vi "EditorMethod runPyProcess.vi"(5 "replace?(T)":bool=TRUE, 7 "func":T1, 8 "error in (no error)":errorcluster, 10 "newScriptCode":string, 11 "dataParam":T3) -> (0 "error out":errorcluster={"status"=FALSE, "code"=0, "source"="codeError source : \ncodeError message : \ncodeError line : "}, 2 "pyCode":string, 3 "newSigInfo":T2, 4 "showMsg":string[](array[string]))   [LabVIEW 2018]
uses:
  ctl/editScriptState.ctl
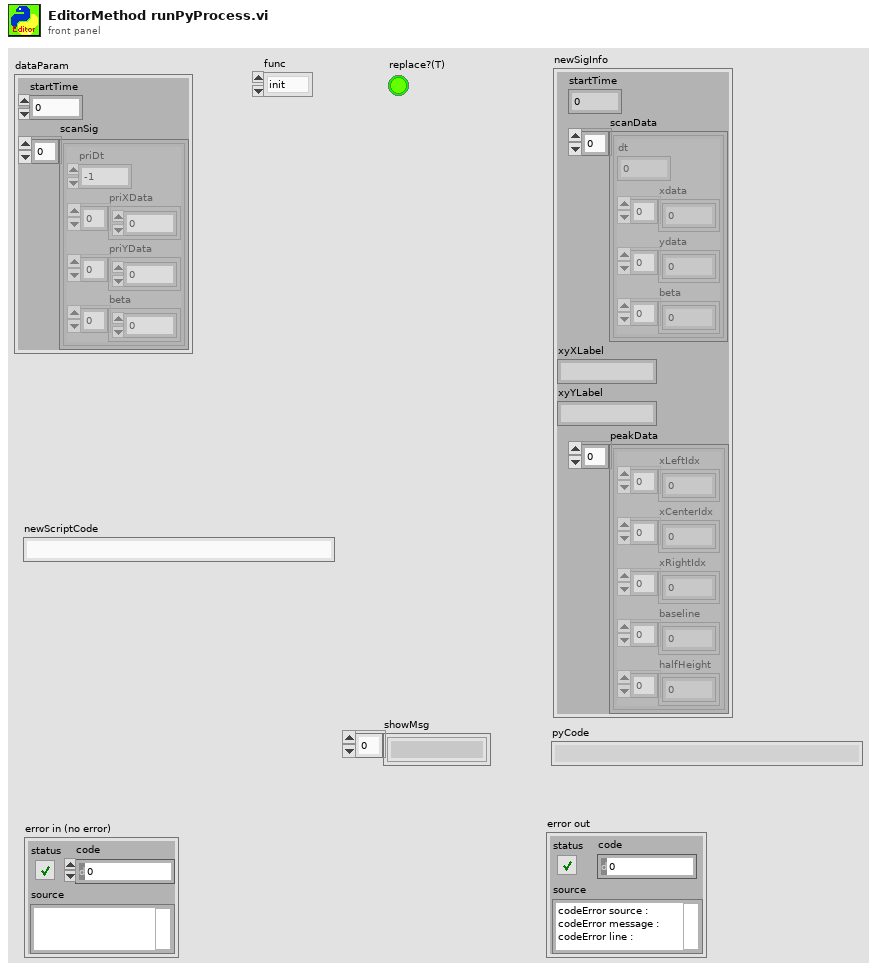
[diagram p1: front panel]
types:
  T1 = typedef "editScriptState.ctl" = enum16{"init", "loadScript", "newScript", "runScript", "close"}
  T2 = cluster{"startTime":dbl, "scanData":cluster{"dt":dbl, "xdata":dbl[], "ydata":sgl[], "beta":dbl[]}[], "xyXLabel":string, "xyYLabel":string, "peakData":cluster{"xLeftIdx":u32[], "xCenterIdx":u32[], "xRightIdx":u32[], "baseline":sgl[], "halfHeight":dbl[]}[]}
  T3 = cluster{"startTime":dbl, "scanSig":cluster{"priDt":dbl, "priXData":dbl[], "priYData":sgl[], "beta":dbl[]}[]}
  T4 = enum16{"open", "replace", "create", "open or create", "replace or create", "replace or create with confirmation"}
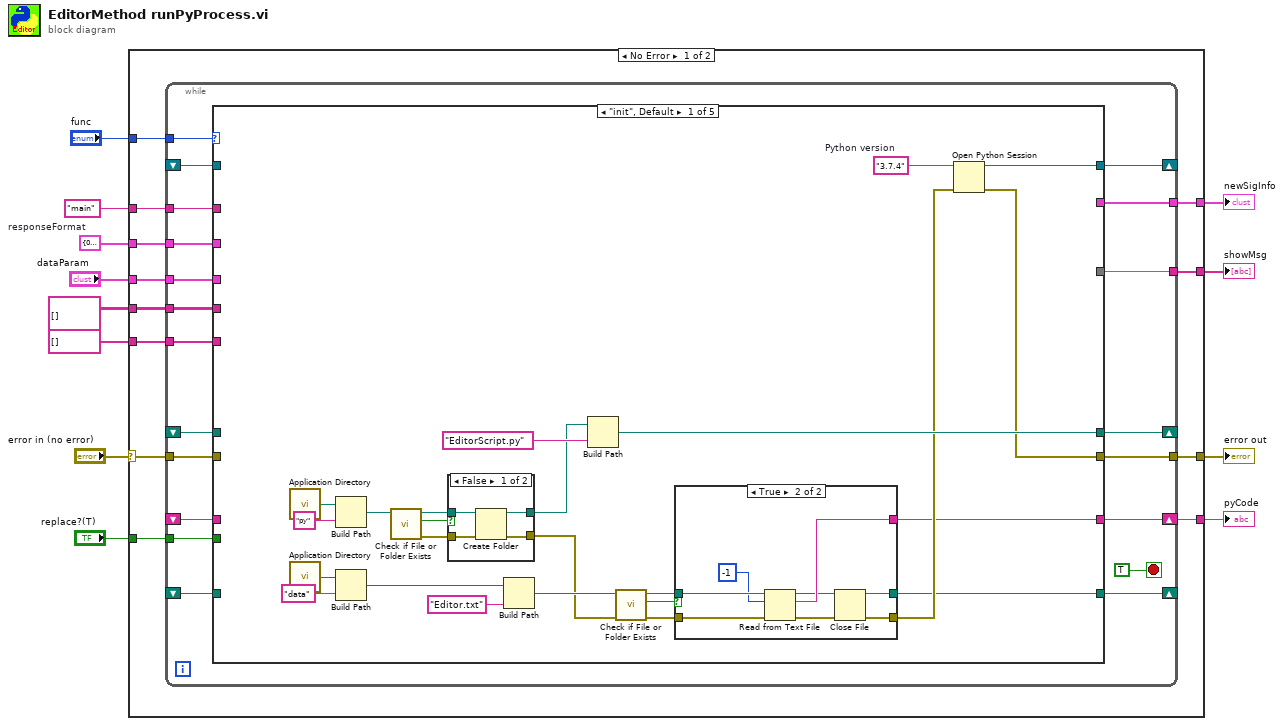
[diagram p0: block diagram]
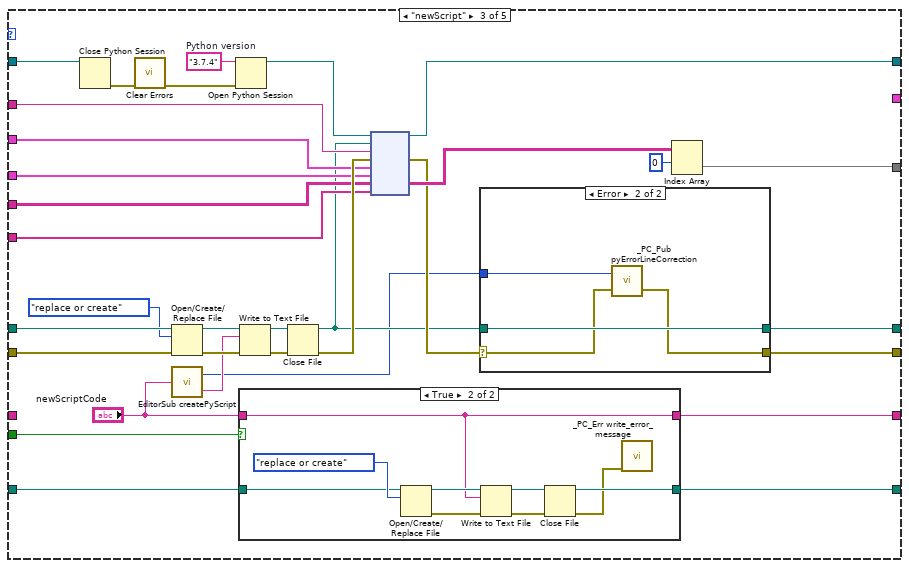
[diagram p5: hidden frame]
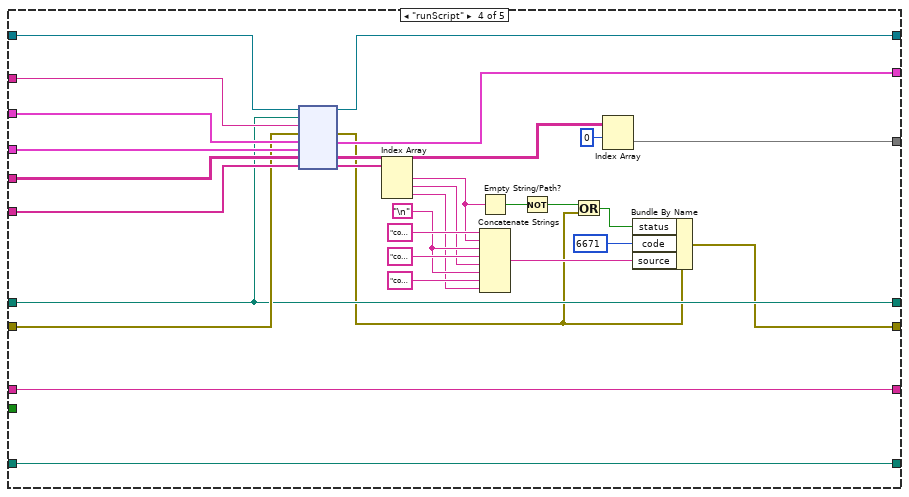
[diagram p8: hidden frame]
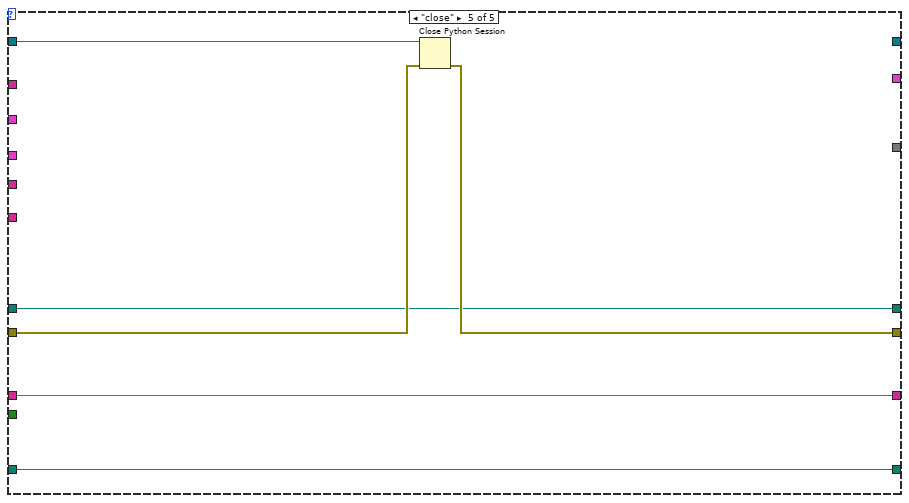
[diagram p9: hidden frame]
diagram:
  w3 = T2 {"startTime"=0.0, "scanData"=[], "xyXLabel"="", "xyYLabel"="", "peakData"=[]}  # responseFormat
  n1 = case shown="No Error" "error in (no error)" {
    selector: "error in (no error)" -> [w19 w176]
    tunnel: "func" -> [w24 _]
    tunnel: [w23 _] -> w12
    tunnel: [w22 _] -> w2
    tunnel: [w21 w176] -> w11
    tunnel: "dataParam" -> [w20 _]
    tunnel: "replace?(T)" -> [w18 _]
    tunnel: [w17 _] -> w7
    tunnel: w3 -> [w16 _]
    tunnel: string[][] [] -> [w15 _]
    tunnel: string[] [] -> [w14 _]
    tunnel: "main" ("function name") -> [w13 _]
    frame No Error {
      n2 = while {
        tunnel: w24 -> [w44]
        shift-right: [w43] -> _
        shift-left: _ -> [w42]
        shift-right: [w41] -> _
        shift-left: _ -> [w40]
        tunnel: [w37] -> w22
        tunnel: w19 -> [w39]
        tunnel: [w35] -> w21
        tunnel: w20 -> [w34]
        tunnel: w18 -> [w33]
        tunnel: [w32] -> w17
        shift-right: [w38] -> w23
        shift-left: _ -> [w31]
        shift-right: [w30] -> _
        shift-left: _ -> [w29]
        tunnel: w16 -> [w28]
        tunnel: w15 -> [w27]
        tunnel: w14 -> [w26]
        tunnel: w13 -> [w25]
        stop <- TRUE stop-if-true
        n3 = case shown="\"init\", Default" w44 {
          tunnel: [w67 w89 w115 w169 _] -> w43
          tunnel: w42 -> [_ w89 w112 w160 w175]
          tunnel: [w58 w86 w93 w147 w173] -> w35
          tunnel: [w59 w88 w94 w148 w172] -> w41
          tunnel: w40 -> [_ w88 w121 w148 w172]
          tunnel: w39 -> [_ w86 w120 w149 w174]
          tunnel: [w45 w87 w122 w155 w170] -> w38
          tunnel: [_ _ _ w162 _] -> w37
          tunnel: w34 -> [_ _ w101 w161 _]
          tunnel: w33 -> [_ _ w113 _ _]
          tunnel: [_ _ w96 w157 _] -> w32
          tunnel: w31 -> [_ w87 _ w155 w170]
          tunnel: [w46 w85 w105 w154 w171] -> w30
          tunnel: w29 -> [_ w85 w106 w154 w171]
          tunnel: w28 -> [_ _ w102 w153 _]
          tunnel: w27 -> [_ _ w100 w151 _]
          tunnel: w26 -> [_ _ w99 w150 _]
          tunnel: w25 -> [_ _ w98 w152 _]
          frame "init", Default {
            w68 = "3.7.4"  # Python version
            n4 = call <vilib>:"Application Directory.vi"() -> ("Application Directory"=w65:path)
            n5 = call <vilib>:"Application Directory.vi"() -> ("Application Directory"=w54:path)
            n6 = Build Path(base path=w65, name or relative path="py") -> (appended path=w56:path)
            n7 = Build Path(base path=w54, name or relative path="data") -> (appended path=w53:path)
            n8 = call <vilib>:"Check if File or Folder Exists.vi"("path"=w56) -> ("error out"=w62:errorcluster, "file or folder exists?"=w64:bool, "dup path"=w63:path)  [unwired: 8 in]
            n9 = case shown="False" w64 {
              tunnel: w63 -> [w82 w84]
              tunnel: w62 -> [w81 w83]
              tunnel: [w80 w84] -> w60
              tunnel: [w79 w83] -> w48
              frame False {
                n10 = Create Folder(path (use dialog)=w82, error in=w81) -> (created path=w80:path, error out=w79:errorcluster)  [unwired: 1 in, 1 out]
              }
              frame True {
              }
            }
            n11 = Build Path(base path=w53, name or relative path="Editor.txt") -> (appended path=w49:path)
            n12 = Build Path(base path=w60, name or relative path="EditorScript.py") -> (appended path=w59:path)
            n13 = call <vilib>:"Check if File or Folder Exists.vi"("error in (no error)"=w48, "path"=w49) -> ("error out"=w50:errorcluster, "file or folder exists?"=w51:bool, "dup path"=w52:path)  [unwired: 7 in]
            n14 = case shown="True" w51 {
              tunnel: w52 -> [w70 w78]
              tunnel: w50 -> [w69 w77]
              tunnel: [_ w76] -> w45
              tunnel: [w70 w72] -> w46
              tunnel: [w69 w71] -> w47
              frame False {
              }
              frame True {
                n15 = Read from Text File(file (use dialog)=w78, count=-1, error in=w77) -> (refnum out=w73:refnum<file>, text=w76:string, error out=w74:errorcluster)  [unwired: 1 in, 1 out]
                n16 = Close File(refnum=w73, error in=w74) -> (path=w72:path, error out=w71:errorcluster)
              }
            }
            n17 = Open Python Session(python version=w68, 3:w47) -> (session out=w67:refnum<k35>, error out=w58:errorcluster)  [unwired: 1 in]
          }
          frame "loadScript" {
          }
          frame "newScript" {
            w109 = "3.7.4"  # Python version
            n18 = Close Python Session(session in=w112) -> (11:w111:errorcluster)  [unwired: 1 in]
            n19 = call <vilib>:"Clear Errors.vi"("error in (no error)"=w111) -> ("error out"=w110:errorcluster)  [unwired: 5 in, 1 out]
            n20 = Open/Create/Replace File(file path (use dialog)=w121, error in=w120, operation (0:open)=T4."replace or create") -> (refnum out=w119:refnum<file>, error out=w118:errorcluster)  [unwired: 3 in, 1 out]
            n21 = call "EditorSub createPyScript.vi"("newScriptCode"="newScriptCode") -> ("scriptStartIdx"=w90:i32, "pyCode"=w103:string)
            n22 = Open Python Session(python version=w109, 3:w110) -> (session out=w108:refnum<k35>)  [unwired: 1 in, 1 out]
            n23 = case shown="True" w113 {
              tunnel: "newScriptCode" -> [w130 w132]
              tunnel: [w130 w132] -> w122
              tunnel: w106 -> [w129 w134]
              tunnel: [w129 w133] -> w105
              frame False {
              }
              frame True {
                n24 = Open/Create/Replace File(file path (use dialog)=w134, operation (0:open)=T4."replace or create") -> (refnum out=w136:refnum<file>, error out=w138:errorcluster)  [unwired: 4 in, 1 out]
                n25 = Write to Text File(file (use dialog)=w136, text=w132, error in=w138) -> (refnum out=w137:refnum<file>, error out=w139:errorcluster)  [unwired: 1 in, 1 out]
                n26 = Close File(refnum=w137, error in=w139) -> (path=w133:path, error out=w131:errorcluster)
                n27 = call "_PC_Err write_error_message.vi"("error in"=w131) -> ()  [unwired: 10 in, 1 out]
              }
            }
            n28 = Write to Text File(file (use dialog)=w119, text=w103, error in=w118) -> (refnum out=w117:refnum<file>, error out=w116:errorcluster)  [unwired: 1 in, 1 out]
            n29 = Close File(refnum=w117, error in=w116) -> (path=w91:path, error out=w107:errorcluster)
            n30 = node(w108, w91, w98, w107, w102, w101, w100, w99) -> (w115:refnum<k35>, w92:errorcluster, w97:string[][])  [unwired: 3 in, 2 out]
            n31 = case shown="Error" w92 {
              selector: w92 -> [w123 w126]
              tunnel: [w124 w128] -> w94
              tunnel: w91 -> [w124 w128]
              tunnel: [w123 w125] -> w93
              tunnel: w90 -> [_ w127]
              frame No Error {
              }
              frame Error {
                n32 = call "_PC_Pub pyErrorLineCorrection.vi"("error in (no error)"=w126, "scriptStartIdx"=w127) -> ("error out"=w125:errorcluster)  [unwired: 1 in]
              }
            }
            n33 = Index Array(array=w97, index (row)=0) -> (element=w96:string[])  [unwired: 1 in]
          }
          frame "runScript" {
            w166 = "\n"
            n34 = node(w160, w148, w152, w149, w153, w161, w151, w150) -> (w169:refnum<k35>, w141:errorcluster, w162:T2, w158:string[][], w159:string[])  [unwired: 1 in, 2 out]
            n35 = Index Array(array=w159) -> (element #1=w144:string, element #2=w164:string, element #3=w163:string)  [unwired: 3 in]
            n36 = Empty String/Path?(string/path=w144) -> (empty?=w143:bool)
            n37 = Concatenate Strings("codeError source : ", w144, w166, "codeError message : ", w164, w166, "codeError line : ", w163) -> (w146:string)
            n38 = Not(x=w143) -> (.not. x?=w142:bool)
            n39 = Or(x=w142, y=w141) -> (x .or. y?=w140:bool)
            n40 = Index Array(array=w158, index (row)=0) -> (element=w157:string[])  [unwired: 1 in]
            n41 = Bundle By Name(cluster=w141, "status"=w140, "code"=6671, "source"=w146) -> (w147:errorcluster)
          }
          frame "close" {
            n42 = Close Python Session(session in=w175, error in=w174) -> (11:w173:errorcluster)
          }
        }
      }
    }
    frame Error {
    }
  }
  "error out" <- w11
  "pyCode" <- w12
  "showMsg" <- w7
  "newSigInfo" <- w2
